vi "ExDebugOpen.vi"() -> ()   [LabVIEW 2010]
uses:
  GlobalSpectHdl.vi
panel:
  out "Camera Open":bool
  out "Spectrometer Open":bool
  in  "Open Spectrometer":bool
  out "error out":errorcluster
  in  "error in (no error)":errorcluster
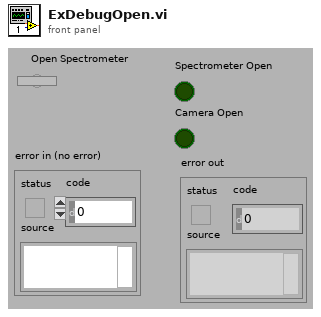
[diagram p1: front panel]
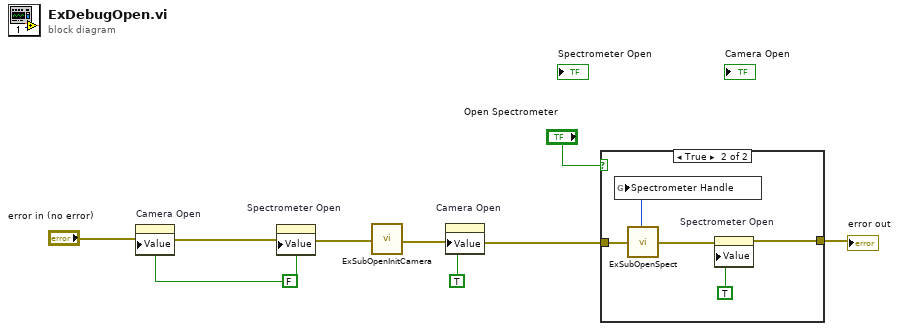
[diagram p0: block diagram]
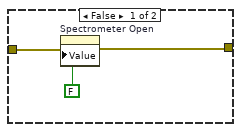
[diagram p2: hidden frame]
diagram:
  w2 = FALSE
  n1 = property on="Camera Open" class="Bool (strict)"(error in="error in (no error)", "Value"=w2) -> (error out=w6:errorcluster)  [unwired: 1 in, 1 out]
  n2 = property on="Spectrometer Open" class="Bool (strict)"(error in=w6, "Value"=w2) -> (error out=w5:errorcluster)  [unwired: 1 in, 1 out]
  n3 = call "ExSubOpenInitCamera.vi"("error in (no error)"=w5) -> ("error out"=w3:errorcluster)  [unwired: 1 out]
  n4 = property on="Camera Open" class="Bool (strict)"(error in=w3, "Value"=TRUE) -> (error out=w4:errorcluster)  [unwired: 1 in, 1 out]
  n5 = case shown="True" "Open Spectrometer" {
    tunnel: w4 -> [w12 w17]
    tunnel: [w11 w15] -> w8
    frame False {
      n6 = property on="Spectrometer Open" class="Bool (strict)"(error in=w12, "Value"=FALSE) -> (error out=w11:errorcluster)  [unwired: 1 in, 1 out]
    }
    frame True {
      n7 = call "ExSubOpenSpect.vi"("error in (no error)"=w17) -> ("Spectromete Handle"=w13:u32, "error out"=w14:errorcluster)
      n8 = global write "GlobalSpectHdl.vi" "Spectrometer Handle"(w13) -> ()
      n9 = property on="Spectrometer Open" class="Bool (strict)"(error in=w14, "Value"=TRUE) -> (error out=w15:errorcluster)  [unwired: 1 in, 1 out]
    }
  }
  "error out" <- w8
